vi "Constructor.vi"(8 "error in (no error)":errorcluster, 11 "ModelDuck in":refnum<class "ModelDuck.lvclass">) -> (0 "error out":errorcluster, 3 "ModelDuck out":refnum<class "ModelDuck.lvclass">)   [LabVIEW 2013, in "ModelDuck.lvclass"]
uses:
  ModelDuck.lvclass
  FlyRocketPowered/FlyRocketPowered.lvclass
  MuteQuack/MuteQuack.lvclass
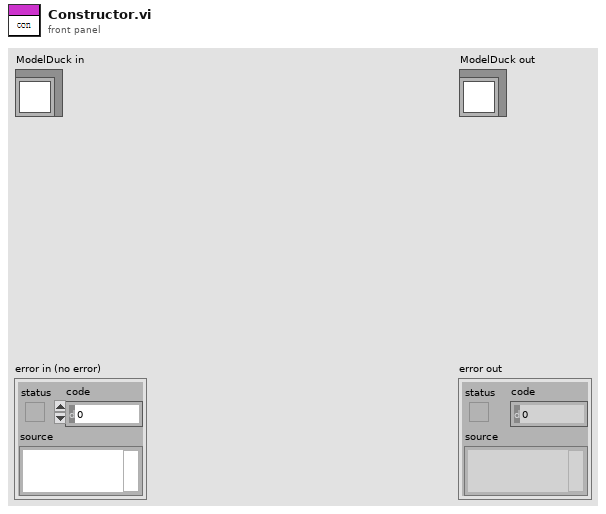
[diagram p1: front panel]
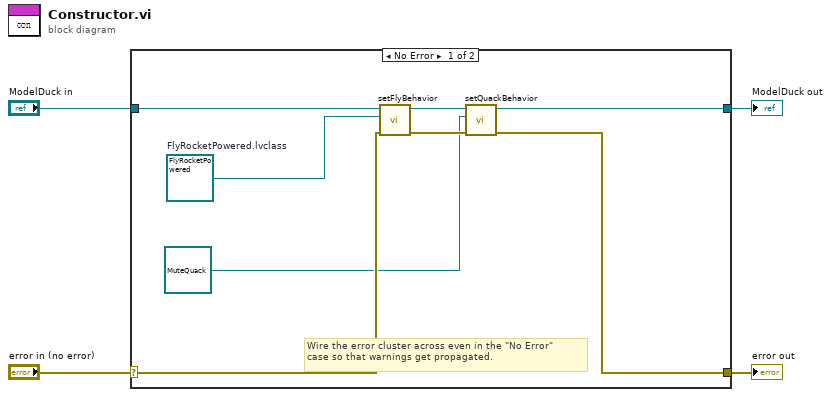
[diagram p0: block diagram]
diagram:
  n1 = case shown="No Error" "error in (no error)" {
    selector: "error in (no error)" -> [w8 w14]
    tunnel: [w7 w14] -> w3
    tunnel: [w10 w13] -> w1
    tunnel: "ModelDuck in" -> [w11 w13]
    frame No Error {
      w6 = refnum<class "FlyRocketPowered.lvclass"> refnum  # FlyRocketPowered.lvclass
      # "Wire the error cluster across even in the \"No Error\"\ncase so that warnings get propagated."
      n2 = call-dynamic "setFlyBehavior.vi"("error in (no error)"=w8, "FlyBehavior.lvclass"=w6, "Duck in"=w11) -> ("error out"=w9:errorcluster, "Duck out"=w12:refnum<class "ModelDuck.lvclass">)  [unwired: 7 in]
      n3 = call-dynamic "setQuackBehavior.vi"("error in (no error)"=w9, "QuackBehavior.lvclass"=refnum<class "MuteQuack.lvclass"> refnum ("MuteQuack.lvclass"), "Duck in"=w12) -> ("error out"=w7:errorcluster, "Duck out"=w10:refnum<class "ModelDuck.lvclass">)  [unwired: 7 in]
    }
    frame Error {
    }
  }
  "error out" <- w3
  "ModelDuck out" <- w1
